vi "HzToTicks.vi"(10 "Duty Cycle":dbl, 11 "Frequency":dbl) -> (3 "Ticks":cluster{"Low Ticks":u32, "High Ticks":u32}={"Low Ticks"=37, "High Ticks"=13})   [LabVIEW 2013, in "PWM Engine.lvlib"]
uses:
  PWM Engine.lvlib
  Shared/Types/PWM.ctl
  Shared/PWM Shared.lvlib
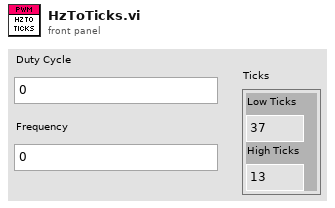
[diagram p1: front panel]
types:
  T1 = typedef "PWM Shared.lvlib/PWM.ctl" = cluster{"Low Ticks":u32, "High Ticks":u32}
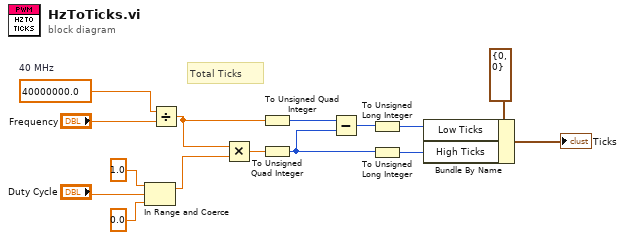
[diagram p0: block diagram]
diagram:
  w15 = 40000000.0  # 40 MHz
  # "Total Ticks"
  n1 = In Range and Coerce(upper limit=1.0, x="Duty Cycle", lower limit=0.0) -> (coerced(x)=w10:dbl)  [unwired: 1 out]
  n2 = Divide(x=w15, y="Frequency") -> (x/y=w5:dbl)
  n3 = Multiply(x=w5, y=w10) -> (x*y=w7:dbl)
  n4 = To Unsigned Quad Integer(1:w5) -> (0:w9:u64)
  n5 = To Unsigned Quad Integer(1:w7) -> (0:w6:u64)
  n6 = Subtract(x=w9, y=w6) -> (x-y=w8:u64)
  n7 = To Unsigned Long Integer(number=w8) -> (unsigned 32bit integer=w4:u32)
  n8 = To Unsigned Long Integer(number=w6) -> (unsigned 32bit integer=w1:u32)
  n9 = Bundle By Name(cluster=T1 {"Low Ticks"=0, "High Ticks"=0} ("Ticks"), "Low Ticks"=w4, "High Ticks"=w1) -> (→"Ticks":T1)
